vi "XY Graph Show Plot.vi"(7 "Hide All Other Plots (F)":bool, 8 "error in (no error)":errorcluster, 10 "Selected Plot Index":i32, 11 "XYGraph in":T1) -> (0 "error out":errorcluster, 3 "XYGraph out":T1)   [LabVIEW 2021, in "XY Graph Add-Ons.lvlib"]
uses:
  XY Graph Add-Ons.lvlib
  XY Graph Refnum.ctl
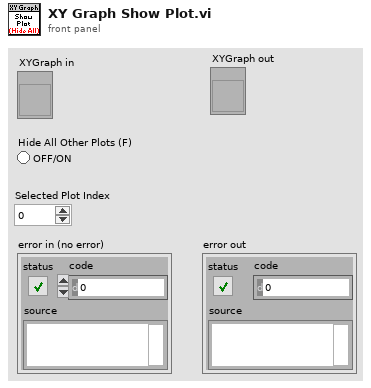
[diagram p1: front panel]
types:
  T1 = typedef "XY Graph Add-Ons.lvlib/XY Graph Refnum.ctl" = refnum<vi>
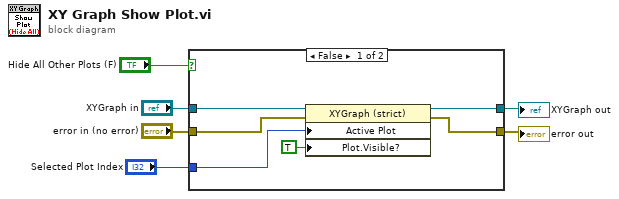
[diagram p0: block diagram]
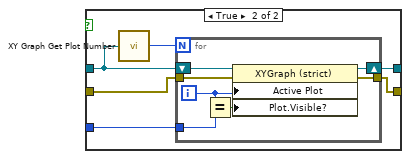
[diagram p2: hidden frame]
diagram:
  n1 = case shown="False" "Hide All Other Plots (F)" {
    tunnel: "XYGraph in" -> [w12 w14]
    tunnel: [w10 w15] -> w6
    tunnel: "error in (no error)" -> [w11 w17]
    tunnel: [w7 w16] -> w5
    tunnel: "Selected Plot Index" -> [w9 w18]
    frame False {
      n2 = property class="XYGraph (strict)"(reference=w12, error in=w11, "Active Plot"=w9, "Plot.Visible?"=TRUE ("Plot.Visible")) -> (reference out=w10:T1, error out=w7:errorcluster)
    }
    frame True {
      n3 = call "XY Graph Get Plot Number.vi"("XYGraph"=w14) -> ("# Plots"=w13:i32)  [unwired: 8 in]
      n4 = for {
        N: w13 -> [_]
        tunnel: w18 -> [w25]
        tunnel: w17 -> [w23]
        tunnel: [w22] -> w16
        shift-right: [w21] -> w15
        shift-left: w14 -> [w24]
        i -> [w20]
        n5 = Equal?(x=w20, y=w25) -> (x = y?=w19:bool)
        n6 = property class="XYGraph (strict)"(reference=w24, error in=w23, "Active Plot"=w20, "Plot.Visible?"=w19) -> (reference out=w21:T1, error out=w22:errorcluster)
      }
    }
  }
  "XYGraph out" <- w6
  "error out" <- w5
